vi "NI VeriStand - Get Target Operating System.vi"(8 "error in (no error)":errorcluster, 11 "Item Ref in":T1 format="%.0x") -> (0 "error out":errorcluster, 2 "Operating System Name":string, 3 "Item Ref out":T1 format="%.0x")   [LabVIEW 2015]
uses:
  <vilib>/NI Veristand/Custom Device API/Custom Device Item Ref.ctl
  NationalInstruments.VeriStand.SystemStorage
  <vilib>/NI VeriStand/Custom Device Tools/Custom Device Utility Library/Custom Device Utility Library.lvlib
  <vilib>/NI VeriStand/Custom Device API/Custom Device API.lvlib
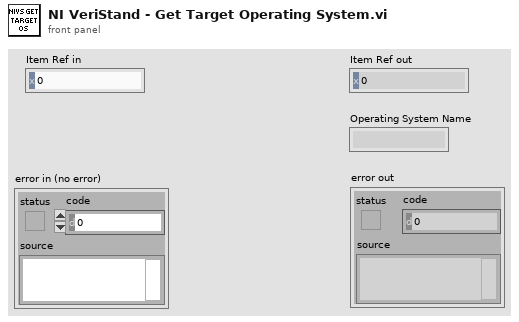
[diagram p1: front panel]
types:
  T1 = typedef "Custom Device API.lvlib/Custom Device Item Ref.ctl" = u64
  T2 = typedef "Custom Device API.lvlib/Custom Device Pointer.ctl" = refnum<k24>
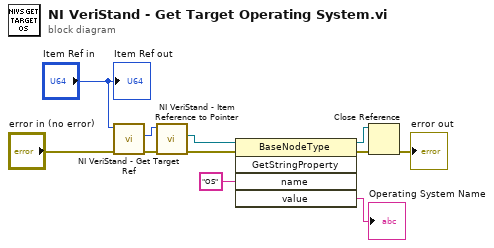
[diagram p0: block diagram]
diagram:
  n1 = call <vilib>:"NI VeriStand - Get Target Ref.vi"("error in"="error in (no error)", "Item Ref in"="Item Ref in") -> ("error out"=w1:errorcluster, "Target Ref"=w11:T1)  [unwired: 6 in, 2 out]
  n2 = call <vilib>:"NI VeriStand - Item Reference to Pointer.vi"("error in (no error)"=w1, "Item Ref in"=w11) -> ("error out"=w10:errorcluster, "Node Pointer"=w9:T2)  [unwired: 6 in, 2 out]
  n3 = invoke class="BaseNodeType" method="GetStringProperty"(reference=w9, error in=w10, "name"="OS") -> (reference out=w8:T2, error out=w7:errorcluster, "value"=→"Operating System Name":string)  [unwired: 2 in, 2 out]
  n4 = Close Reference(reference=w8, error in (no error)=w7) -> (error out=→"error out":errorcluster)
  "Item Ref out" <- "Item Ref in"
